vi "Search for Bad Pointers.vi"(5 "Recurse Up List":bool, 7 "Linked List ID":string, 8 "error in (no error)":errorcluster, 9 "Removed Unique ID":string, 10 "Bad Pointers":string[](array[string]), 11 "Linked List in":refnum<class "Linked List.lvclass">) -> (0 "error out":errorcluster, 2 "IDs":string[](array[string]), 3 "Linked List out":refnum<class "Linked List.lvclass">)   [LabVIEW 2020, in "Linked Lists.lvlib" / "Linked List.lvclass"]
uses:
  <vilib>/gpm_packages/@cs/linked-list/Source/Linked List/Linked List/Linked List.lvclass
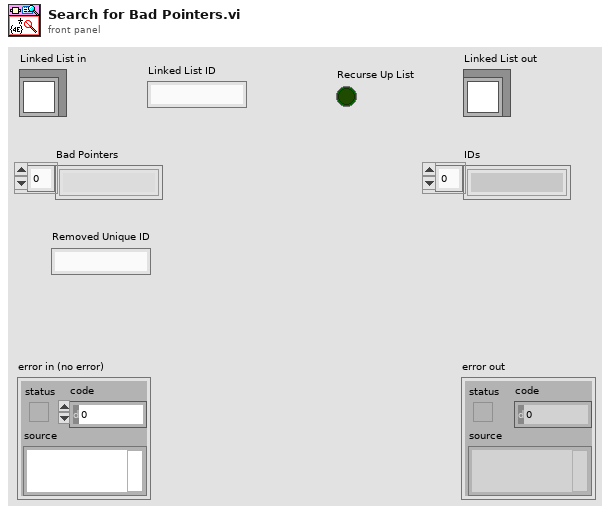
[diagram p1: front panel]
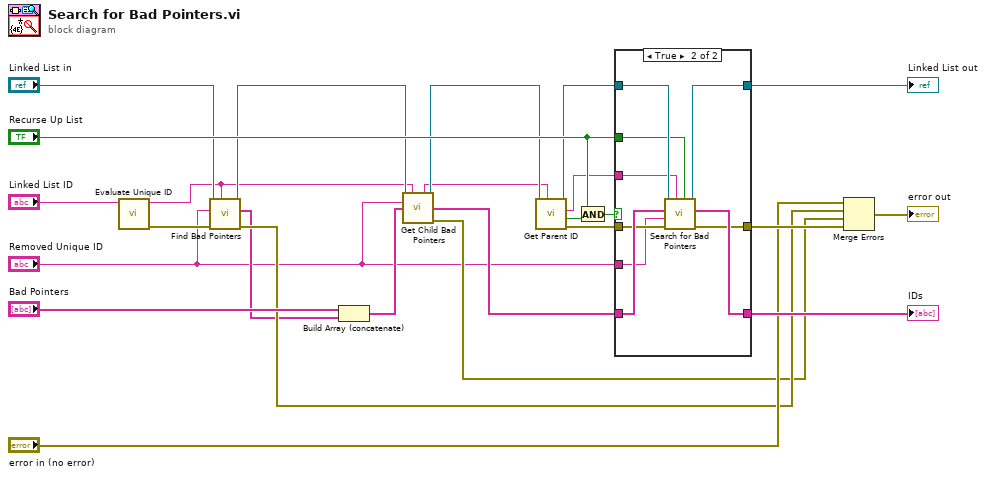
[diagram p0: block diagram]
diagram:
  n1 = call <vilib>:"Evaluate Unique ID.vi"("Unique ID"="Linked List ID") -> ("error out"=w11:errorcluster, "Unique ID Out"=w4:string)  [unwired: 9 in]
  n2 = call <vilib>:"Find Bad Pointers.vi"("Unique ID"=w4, "error in (no error)"=w11, "Removed Unique ID"="Removed Unique ID", "Linked List in"="Linked List in") -> ("error out"=w10:errorcluster, "Bad Pointers"=w9:string[], "Linked List out"=w8:refnum<class "Linked List.lvclass">)  [unwired: 5 in]
  n3 = Build Array (concatenate)("Bad Pointers", w9) -> (w6:string[])
  n4 = call <vilib>:"Get Child Bad Pointers.vi"("Linked List in"=w8, "Linked List ID"=w4, "Removed Unique ID"="Removed Unique ID", "Bad Pointers"=w6) -> ("Linked List ID out"=w3:string, "Linked List out"=w7:refnum<class "Linked List.lvclass">, "Missing GUIDs out"=w2:string[], "error out"=w5:errorcluster)  [unwired: 8 in]
  n5 = call-dynamic "Get Parent ID.vi"("Linked List ID"=w3, "Linked List in"=w7) -> ("error out"=w18:errorcluster, "Valid Parent ID"=w17:bool, "Parent ID"=w16:string, "Linked List out"=w19:refnum<class "Linked List.lvclass">)  [unwired: 6 in]
  n6 = And(x="Recurse Up List", y=w17) -> (x .and. y?=w15:bool)
  n7 = case shown="True" w15 {
    tunnel: [w27 w30] -> w23
    tunnel: w18 -> [w27 w31]
    tunnel: w19 -> [w28 w37]
    tunnel: [w28 w36] -> w24
    tunnel: [w26 w32] -> w22
    tunnel: w2 -> [w26 w33]
    tunnel: w16 -> [_ w35]
    tunnel: "Recurse Up List" -> [_ w34]
    tunnel: "Removed Unique ID" -> [_ w29]
    frame False {
    }
    frame True {
      n8 = call-dynamic "Search for Bad Pointers.vi"("Recurse Up List"=w34, "Linked List ID"=w35, "error in (no error)"=w31, "Removed Unique ID"=w29, "Bad Pointers"=w33, "Linked List in"=w37) -> ("error out"=w30:errorcluster, "IDs"=w32:string[], "Linked List out"=w36:refnum<class "Linked List.lvclass">)  [unwired: 3 in]
    }
  }
  "Linked List out" <- w24
  "IDs" <- w22
  n9 = Merge Errors("error in (no error)", w10, w5, w23) -> (→"error out":errorcluster)
